vi "Galobal variable_TI.vi"() -> ()   [LabVIEW 2015]
panel:
  in  "Digital Output":bool[](array[boolean])
  in  "Auto Exit":bool
  in  "Slid Servo Home bit":bool
  in  "Call Home M2":bool
  in  "Call Home M1":bool
  in  "Error Message":string
  in  "Barcode Lenght":i32
  in  "Barcode Scan Bit":bool
  in  "Barcode Data":string
  in  "Control Enable":bool
  in  "Stop M1":bool
  in  "Stop M2":bool
  in  "Programlist":string[](array[string])
  out "Errror No.":i32
  in  "STM Done Bit":bool
  in  "Shift":T1={"To-A"=timestamp(3526451999 s since 1904-01-01), "From-A"=timestamp(3526594200 s since 1904-01-01), "From-B"=timestamp(3526452000 s since 1904-01-01), "To-B"=timestamp(3526482599 s since 1904-01-01), "From-C"=timestamp(3526482600 s since 1904-01-01), "To-C"=timestamp(3526421399 s since 1904-01-01), "Shift"=""} {"To-A" format="%<%H:%M:%S\n%d/%m/%Y>T"; "From-A" format="%<%H:%M:%S\n%d/%m/%Y>T"; "From-B" format="%<%H:%M:%S\n%d/%m/%Y>T"; "To-B" format="%<%H:%M:%S\n%d/%m/%Y>T"; "From-C" format="%<%H:%M:%S\n%d/%m/%Y>T"; "To-C" format="%<%H:%M:%S\n%d/%m/%Y>T"}
  in  "Offset_2":dbl
  in  "Offset_1":dbl
  in  "Slop _2":dbl
  in  "Slop_1":dbl
  out "Analoge Input":dbl[](array[numeric])
  out "AI_as DI":bool[](array[boolean])
  out "Manual DO":bool[](array[boolean])
  in  "Manual CMD":bool
  out "File Path":path[](array[path])
  out "Digital input":bool[](array[boolean])
  in  "User Name":string
  in  "Exit":bool
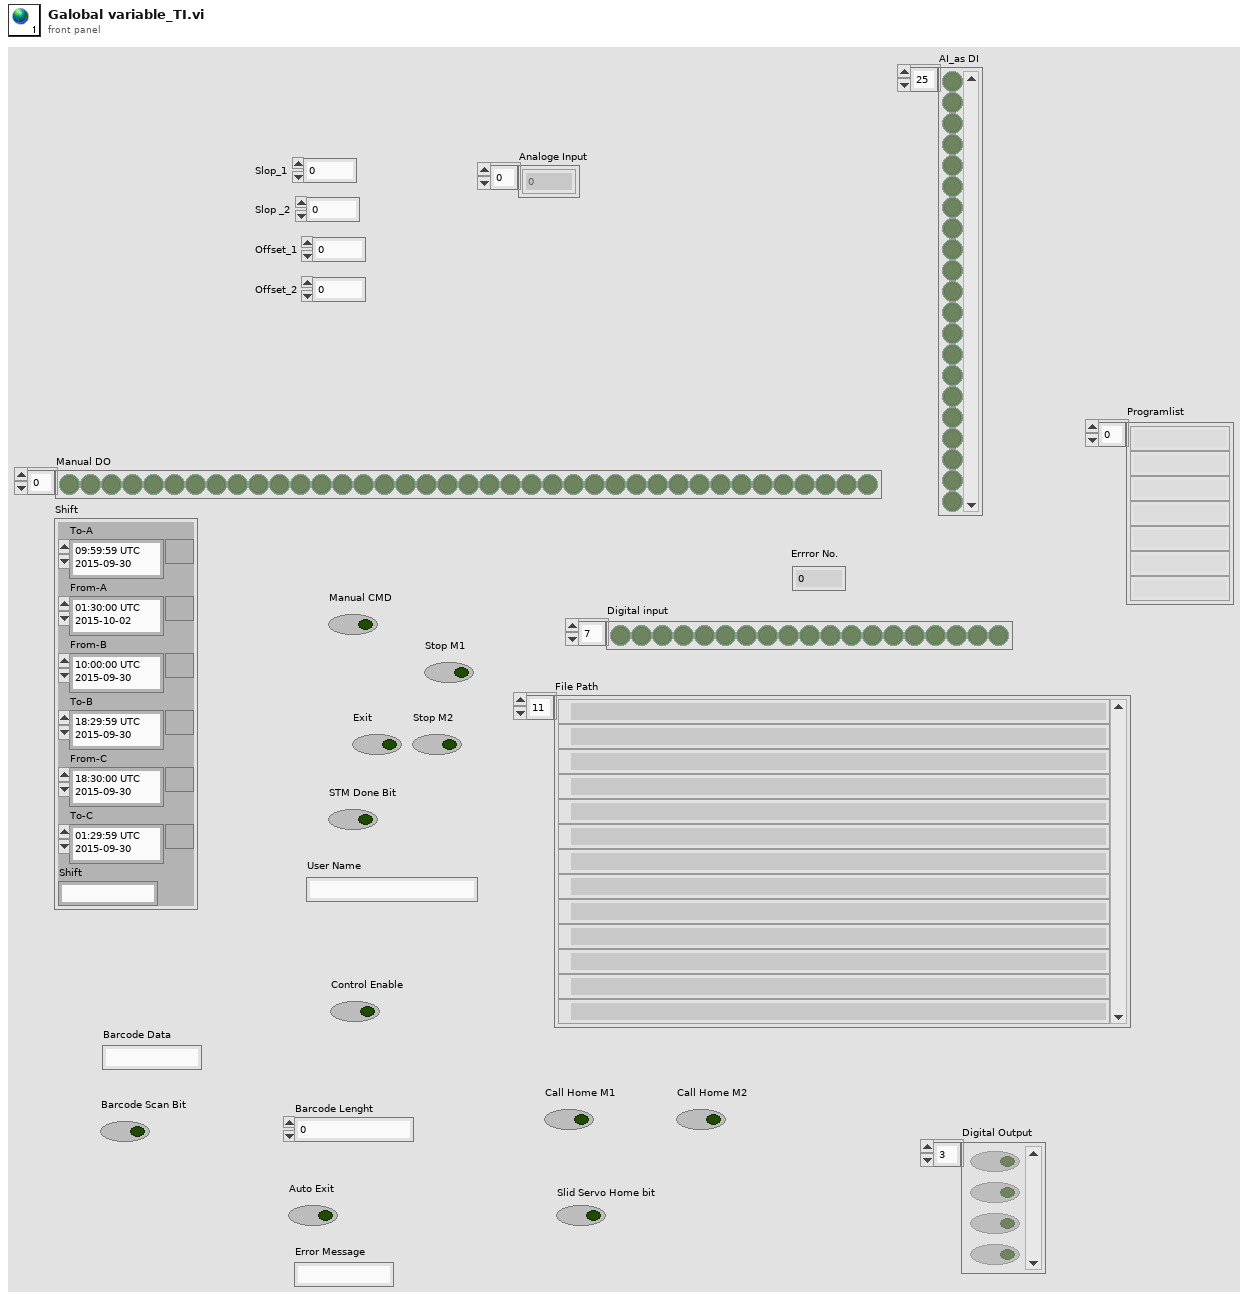
[diagram p1: front panel]
types:
  T1 = cluster{"To-A":timestamp, "From-A":timestamp, "From-B":timestamp, "To-B":timestamp, "From-C":timestamp, "To-C":timestamp, "Shift":string}
diagram:
